vi "BRig_dataRT_stats__nReward_left.vi"() -> (2 "output_nReward_left":i32)   [LabVIEW 2014]
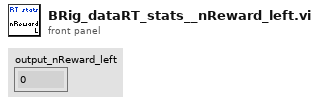
[diagram p1: front panel]
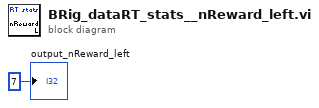
[diagram p0: block diagram]
diagram:
  "output_nReward_left" <- 7 ("output_iBlock")
